vi "Boiler System Open.vi"(8 "error in":errorcluster) -> (0 "error out 2":errorcluster, 2 "Notifiers":T2, 3 "Message Queues out 2":T1, 5 "User Event - Stop 2":refnum<user-event>, 7 "Stop Event Registration Refnum 2":refnum<event-registration>)   [LabVIEW 2015]
uses:
  User Event - Stop/User Event - Stop.lvlib
  Message Queue/Message Queue.lvlib
  Message Queue/Message Cluster.ctl
  Message Queue/All Message Queues.ctl
  Notifiers/Notifiers.ctl
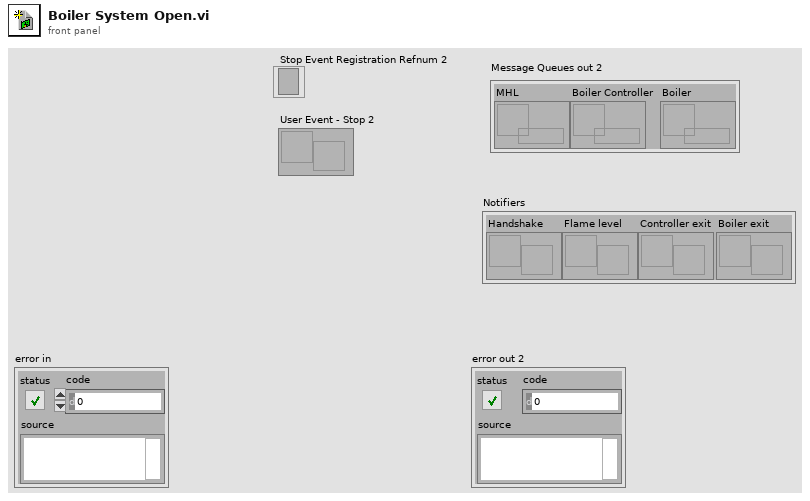
[diagram p1: front panel]
types:
  T1 = typedef "Message Queue.lvlib/All Message Queues.ctl" = cluster{"MHL":refnum<queue>, "Boiler Controller":refnum<queue>, "Boiler":refnum<queue>}
  T2 = typedef "Notifiers.ctl" = cluster{"Handshake":refnum<notifier>, "Flame level":refnum<notifier>, "Controller exit":refnum<notifier>, "Boiler exit":refnum<notifier>}
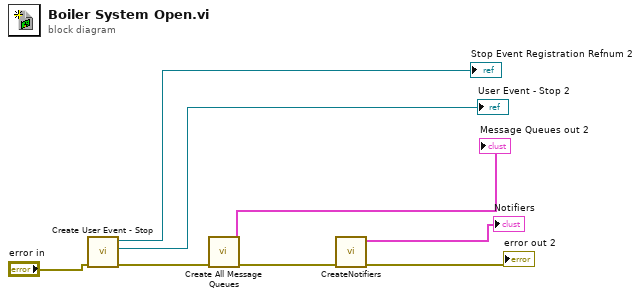
[diagram p0: block diagram]
diagram:
  n1 = call "Create User Event - Stop.vi"("error in (no error)"="error in") -> ("error out"=w6:errorcluster, "User Event - Stop"=→"User Event - Stop 2":refnum<user-event>, "Stop Event Registration Refnum"=→"Stop Event Registration Refnum 2":refnum<event-registration>)  [unwired: 8 in]
  n2 = call "Create All Message Queues.vi"("error in"=w6) -> ("error out"=w5:errorcluster, "Message Queues out"=→"Message Queues out 2":T1)  [unwired: 9 in]
  n3 = call "CreateNotifiers.vi"("error in"=w5) -> ("error out"=→"error out 2":errorcluster, "Notifiers"=→"Notifiers":T2)  [unwired: 9 in]
